vi "预览控件.vi"(8 "error in (no error)":errorcluster caption="错误输入（无错误）", 10 "鼠标位置":T1, 11 "程序响应 输入":refnum<class "程序响应.lvclass">) -> (0 "error out":errorcluster caption="错误输出", 3 "程序响应 输出":refnum<class "程序响应.lvclass">)   [LabVIEW 2018, in "程序响应.lvlib" / "程序响应.lvclass"]
uses:
  <vilib>/Utility/miscctls.llb/LVPoint32TypeDef.ctl
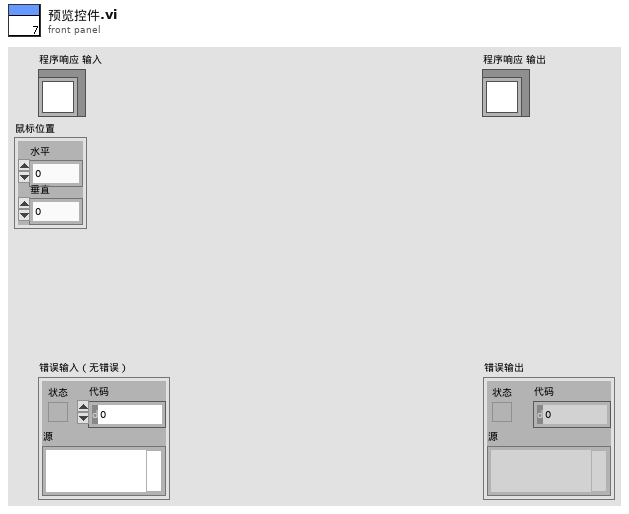
[diagram p1: front panel]
types:
  T1 = typedef "LVPoint32TypeDef.ctl" = cluster{"Horizontal":i32, "Vertical":i32}
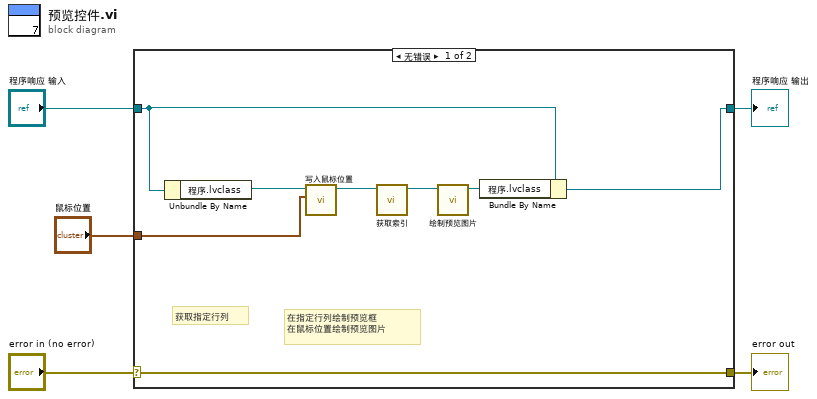
[diagram p0: block diagram]
diagram:
  n1 = case shown="无错误" "error in (no error)" {
    selector: "error in (no error)" -> [w13 w15]
    tunnel: [w13 w15] -> w4
    tunnel: [w10 w14] -> w2
    tunnel: "程序响应 输入" -> [w11 w14]
    tunnel: "鼠标位置" -> [w7 _]
    frame No Error {
      # "在指定行列绘制预览框\n在鼠标位置绘制预览图片"
      # "获取指定行列"
      n2 = Unbundle By Name(w11) -> ("程序.lvclass"=w9:refnum<class "程序.lvclass">)
      n3 = call-dynamic "写入鼠标位置.vi"("Point32"=w7, "程序输入"=w9) -> ("程序输出"=w8:refnum<class "程序.lvclass">)  [unwired: 8 in, 1 out]
      n4 = call-dynamic "获取索引.vi"("程序 输入"=w8) -> ("程序 输出"=w6:refnum<class "程序.lvclass">)  [unwired: 9 in, 1 out]
      n5 = call-dynamic "绘制预览图片.vi"("程序 输入"=w6) -> ("程序 输出"=w12:refnum<class "程序.lvclass">)  [unwired: 9 in, 1 out]
      n6 = Bundle By Name(cluster=w11, "程序.lvclass"=w12) -> (w10:refnum<class "程序响应.lvclass">)
    }
    frame Error {
    }
  }
  "error out" <- w4
  "程序响应 输出" <- w2
